vi "Close.vi"   [LabVIEW 2020, in "SLSC.lvlib"]
doc: "Closes an SLSC session or an open SLSC command/property reference."
uses:
  <vilib>/SLSC/SLSC.lvlib
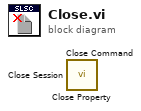
[diagram p0: block diagram]
diagram:
  n1 = call <vilib>:"Close Property.vi"() -> ()  [unwired: 15 in, 1 out]
  n2 = call <vilib>:"Close Command.vi"() -> ()  [unwired: 15 in, 1 out]
  n3 = call <vilib>:"Close Session.vi"() -> ()  [unwired: 15 in, 1 out]
